vi "switch magnet realtime.vi"() -> ()   [LabVIEW 2009]
doc: "This vi sets/recieves values from the switch magnet power supply via fpga"
uses:
  <vilib>/rvi/interface/nirviOpenFPGA/nirviOpenFPGA.xnode
  FPGA Bitfiles/Control software p~3C_FPGA Target 3_switchmagnet_fpga.vi.lvbitx
  switchmagnet_fpga.vi
  <vilib>/FPGAPlugInAG/cRIO-9074/nirviIntfOpen_cRIO-9074.vi
  <vilib>/rvi/interface/nirviReadWriteControl/nirviReadWriteControl.xnode
  <vilib>/LabVIEW Targets/FPGA/RIO/nirio_HostInterface/nirio_ReadBig.vi
  <vilib>/rvi/errors/niLvFpgaAdjustHostInterfaceError.vi
  <vilib>/rvi/interface/common/niFpgaNodeNameForErrorReporting.ctl
  <vilib>/rvi/errors/niLvFpgaWhatHappensToTopLevelVI.ctl
  <vilib>/functionblocks/FB Core/FB Core.xnode
  <vilib>/functionblocks/Control/PID/PID.vi
  <vilib>/LabVIEW Targets/FPGA/RIO/nirio_HostInterface/nirio_WriteBig.vi
  <vilib>/userDefined/High Color/nirio_resource_hc.ctl
  <vilib>/functionblocks/NI_FunctionBlock Libraries.lvlib
panel:
  out "Waveform Chart":dbl(graph)
  in  "stop":bool
  out "unsigned byte array":u8[](array[numeric])
  out "concatenated string":string
  out "error out 2":errorcluster
  in  "proportional gain (Kc) 2":dbl=20.0
  in  "integral time (Ti, min)":dbl=0.01
  in  "derivative time (Td, min)":dbl=0.06
  in  "auto? (T)":bool=TRUE
  out "Serial Loop":i32
  out "setpoint":dbl
  out "abs(x)":dbl
  out "match + rest of string":string
  in  "x":dbl
  out "ps setting":dbl
  out "string":string
  out "Array":u8[](array[numeric])
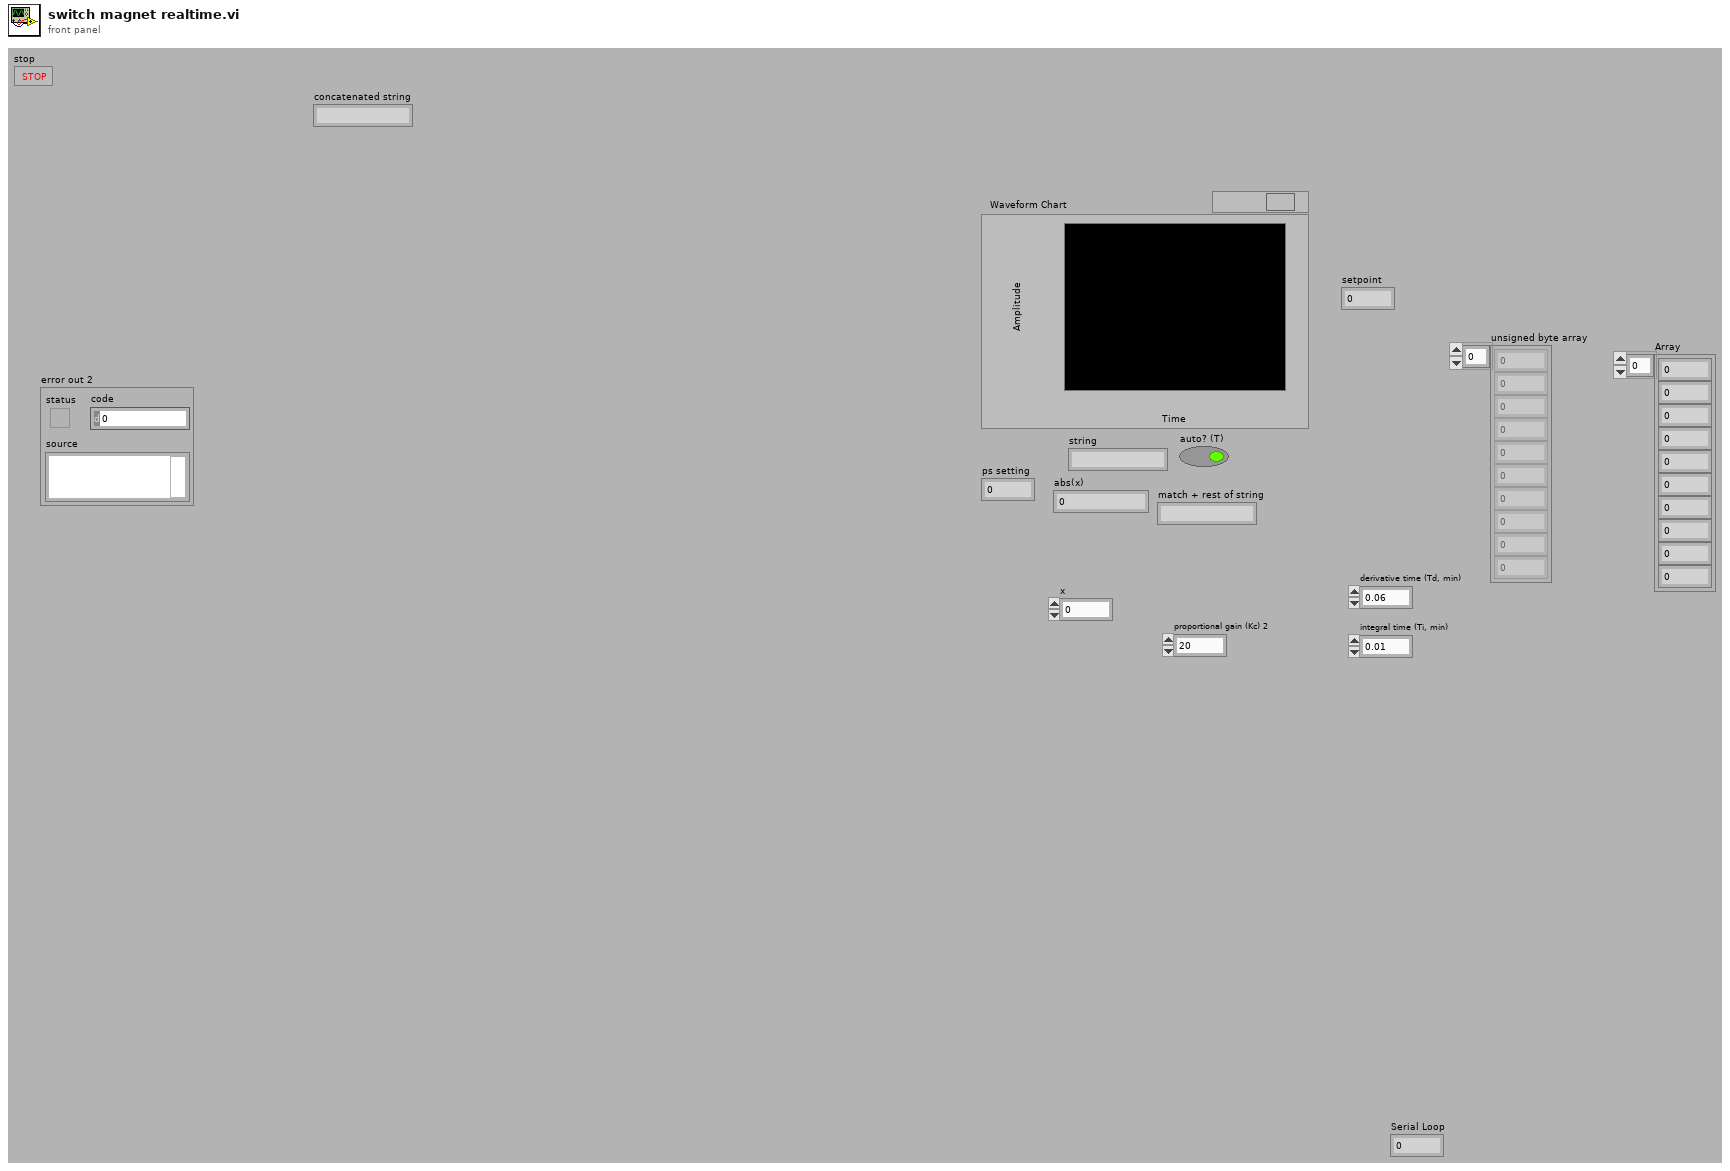
[diagram p1: front panel]
types:
  T1 = typedef "niFpgaNodeNameForErrorReporting.ctl" = enum16{"Open FPGA VI Reference", "Read/Write Control", "Invoke Method: Abort", "Invoke Method: Acknowledge IRQ", "Invoke Method: Download", "Invoke Method: FIFO.Configure", "Invoke Method: FIFO.Read", "Invoke Method: FIFO.Start", "Invoke Method: FIFO.Stop", "Invoke Method: FIFO.Write", "Invoke Method: Reset", "Invoke Method: Run", "Invoke Method: Wait on IRQ", "Close FPGA VI Reference"}
  T2 = typedef "niLvFpgaWhatHappensToTopLevelVI.ctl" = enum16{"top level VI scripted behind XNode", "top level VI inlined behind XNode"}
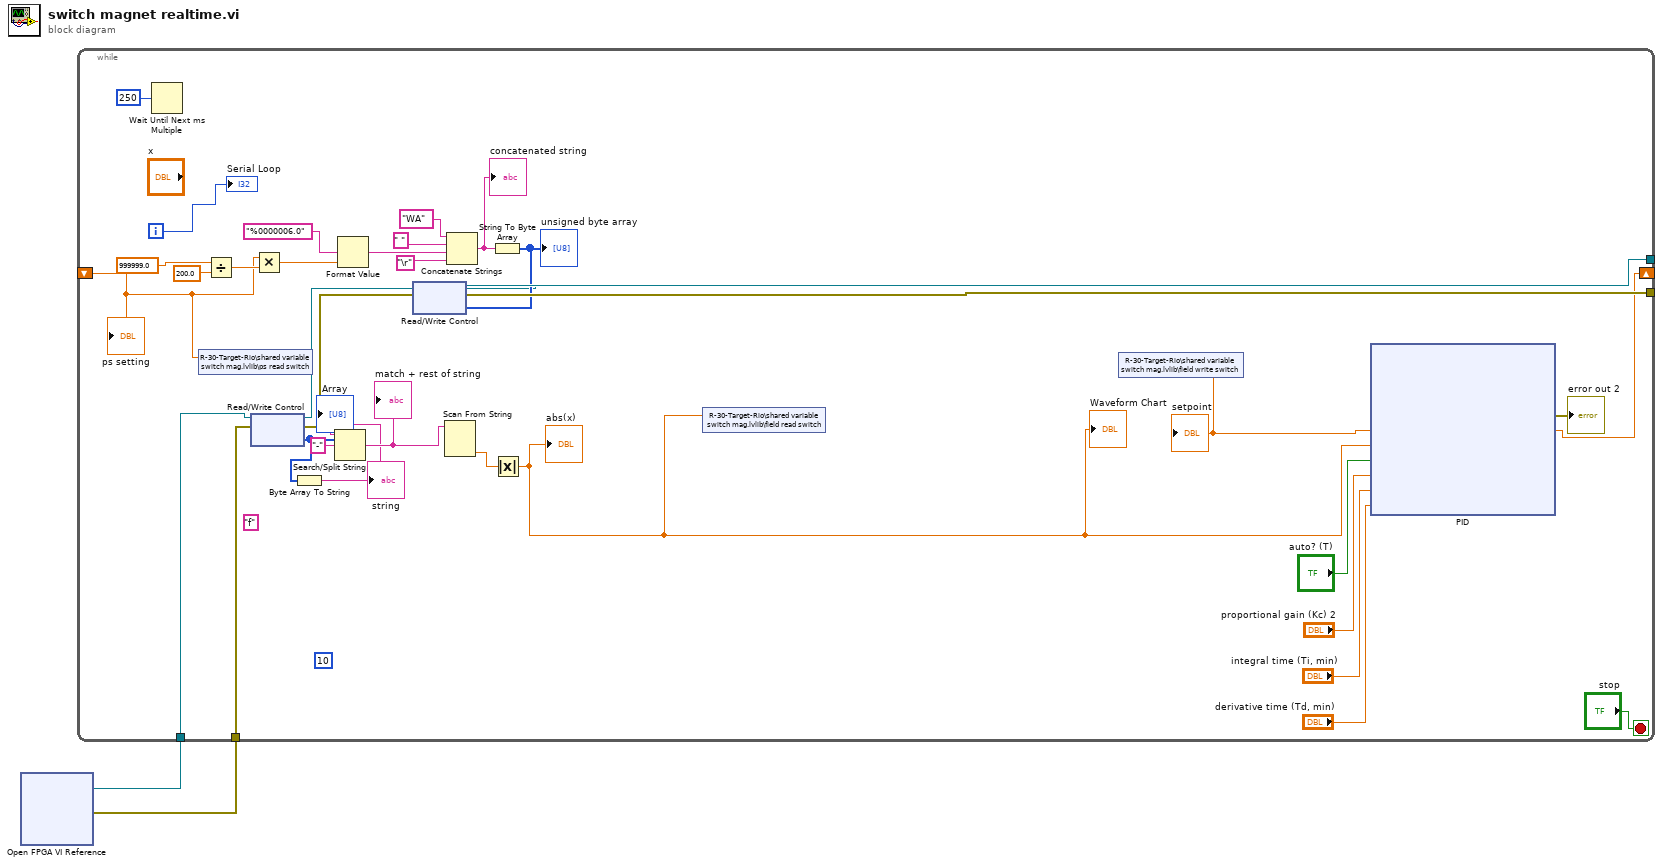
[diagram p0: block diagram]
diagram:
  n1 = xnode "Open FPGA VI Reference"() -> ("FPGA VI Reference Out"=w2:refnum<k20>, "error out"=w1:errorcluster)  [unwired: 2 in]
  n2 = while {
    tunnel: [w25] -> _
    tunnel: [w24] -> _
    shift-right: [w20] -> _
    shift-left: _ -> [w6]
    tunnel: w2 -> [w12]
    tunnel: w1 -> [w10]
    i -> [w15]
    stop <- "stop" stop-if-true
    (unwired) u32 10 ("byte count")
    (unwired) "f" ("write buffer")
    n3 = Wait Until Next ms Multiple(millisecond multiple=u32 250) -> ()  [unwired: 1 out]
    n4 = shared-variable "R-30-Target-Rio\\shared variable switch mag.lvlib\\ps read switch"(w6) -> ()  [unwired: 2 out]
    n5 = Divide(x=999999.0, y=200.0) -> (x/y=w32:dbl)
    n6 = xnode "Read/Write Control"("FPGA VI Reference In"=w12, "error in"=w10) -> ("FPGA VI Reference Out"=w11:refnum<k20>, "error out"=w9:errorcluster, "Array"=w8:u8[])
    "Array" <- w8
    n7 = Multiply(x=w6, y=w32) -> (x*y=w30:dbl)
    n8 = Byte Array To String(unsigned byte array=w8) -> (string=w7:string)
    "string" <- w7
    n9 = Search/Split String(string=w7, search string/char (-)="-") -> (match + rest of string=w13:string)  [unwired: 3 out]
    "match + rest of string" <- w13
    n10 = Format Value(format string="%0000006.0", value (0)=w30) -> (output string=w27:string)  [unwired: 1 out]
    n11 = Scan From String(input string=w13) -> (output 1=w18:dbl)  [unwired: 3 in, 4 out]
    n12 = Concatenate Strings("WA", " ", w27, "\r") -> (w26:string)
    "concatenated string" <- w26
    n13 = String To Byte Array(string=w26) -> (unsigned byte array=w23:u8[])
    "unsigned byte array" <- w23
    n14 = xnode "Read/Write Control"("FPGA VI Reference In"=w11, "error in"=w9, "data 2"=w23) -> ("FPGA VI Reference Out"=w24:refnum<k20>, "error out"=w25:errorcluster)
    n15 = Absolute Value(x=w18) -> (abs(x)=w5:dbl)
    "abs(x)" <- w5
    "Waveform Chart" <- w5
    n16 = shared-variable "R-30-Target-Rio\\shared variable switch mag.lvlib\\field read switch"(w5) -> ()  [unwired: 2 out]
    n17 = shared-variable "R-30-Target-Rio\\shared variable switch mag.lvlib\\field write switch"() -> (w3:dbl)  [unwired: 2 out]
    "setpoint" <- w3
    n18 = xnode "PID"("setpoint"=w3, "process variable"=w5, "auto? (T)"="auto? (T)", "proportional gain (Kc)"="proportional gain (Kc) 2", "integral time (Ti, min)"="integral time (Ti, min)", "derivative time (Td, min)"="derivative time (Td, min)") -> ("error out"=→"error out 2":errorcluster, "output"=w20:dbl)  [unwired: 1 in]
    "Serial Loop" <- w15
    "ps setting" <- w6
  }
